vi "myRIO_BRig_Host_formatData_test2.vi"(7 "input_filePath":string, 8 "input_error":errorcluster, 9 "input_data":u16[][](array[numeric]), 10 "input_headers":string[](array[string]), 11 "input_hdl_Workbooks":refnum<k7>) -> (0 "output_error":errorcluster, 3 "output_hdl_Worksbooks":refnum<k7>)   [LabVIEW 2014]
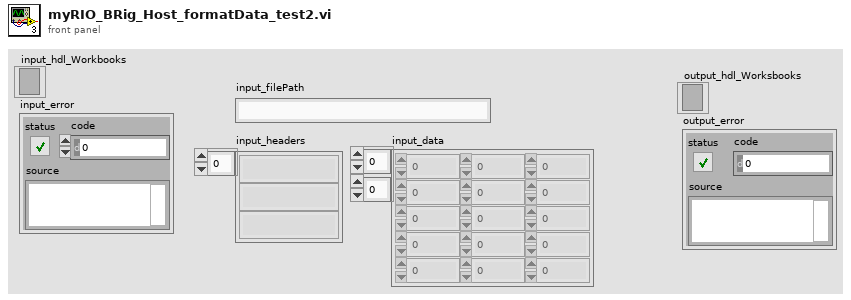
[diagram p1: front panel]
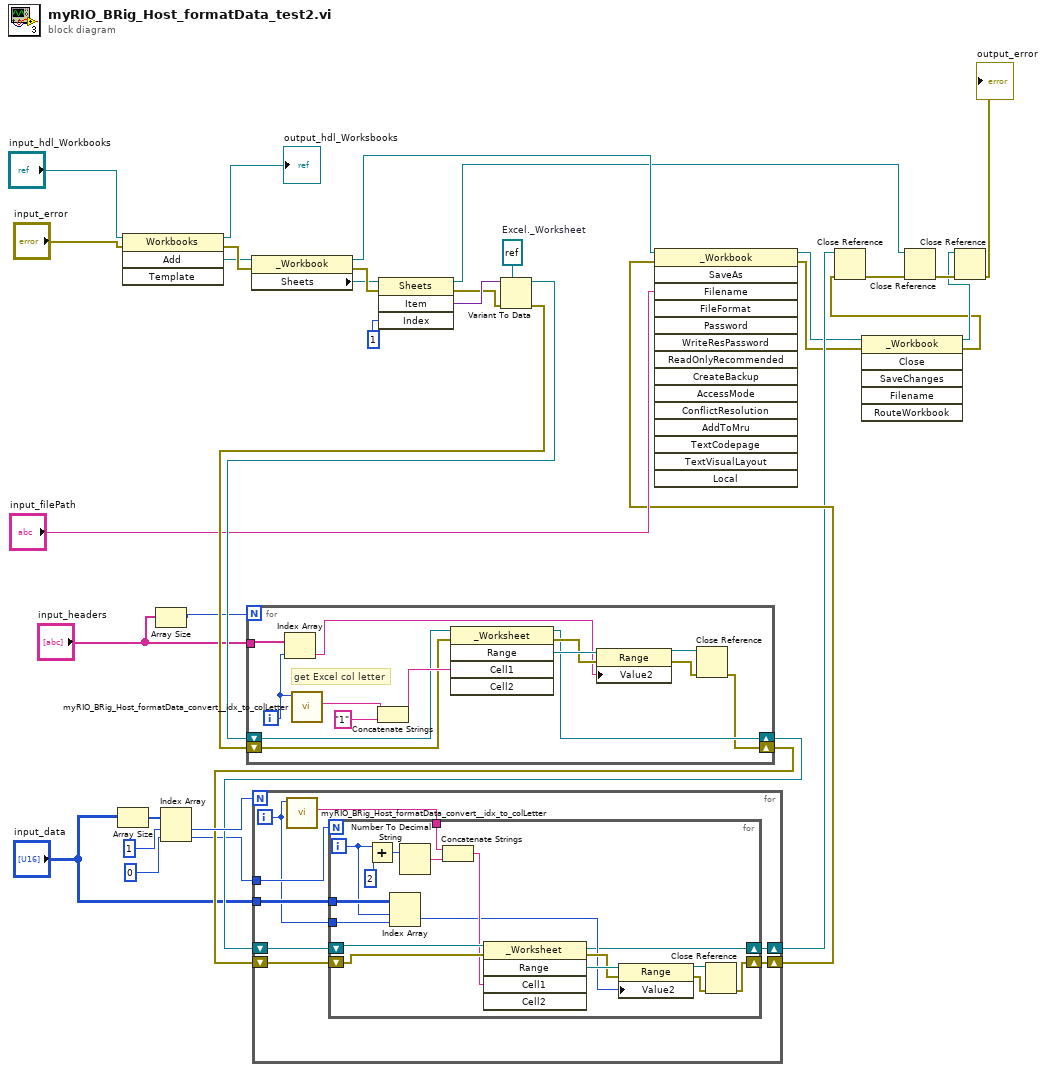
[diagram p0: block diagram]
diagram:
  w30 = refnum<k7> refnum  # Excel._Worksheet
  n1 = Array Size(array="input_data") -> (size(s)=w18:i32[])
  n2 = invoke class="Workbooks" method="Add"(reference="input_hdl_Workbooks", error in="input_error") -> (reference out=→"output_hdl_Worksbooks":refnum<k7>, error out=w34:errorcluster, "Add"=w32:refnum<k7>)  [unwired: 2 in, 1 out]
  n3 = Array Size(array="input_headers") -> (size(s)=w19:i32)
  n4 = Index Array(array=w18, index #1=1 ("index"), index #2=0 ("index")) -> (element #1=w15:i32, element #2=w12:i32)
  n5 = property class="_Workbook"(reference=w32, error in=w34) -> (reference out=w27:refnum<k7>, error out=w35:errorcluster, "Sheets"=w31:refnum<k7>)
  n6 = invoke class="Sheets" method="Item"(reference=w31, error in=w35, "Index"=1) -> (reference out=w26:refnum<k7>, error out=w28:errorcluster, "Item"=w29:variant)  [unwired: 1 in, 1 out]
  n7 = Variant To Data(error in=w28, type=w30, Variant=w29) -> (data=w22:refnum<k7>, error out=w23:errorcluster)
  n8 = for {
    N: w19 -> [_]
    tunnel: "input_headers" -> [w49]
    shift-right: [w39] -> w13
    shift-left: w22 -> [w41]
    shift-right: [w36] -> w14
    shift-left: w23 -> [w40]
    i -> [w48]
    # "get Excel col letter"
    n9 = Index Array(array=w49, index=w48) -> (element=w42:string)
    n10 = call "myRIO_BRig_Host_formatData_convert__idx_to_colLetter.vi"("input_idx"=w48) -> ("output_colLetter"=w46:string)  [unwired: 10 in]
    n11 = Concatenate Strings(w46, "1" ("string")) -> (w45:string)
    n12 = invoke class="_Worksheet" method="Range"(reference=w41, error in=w40, "Cell1"=w45) -> (reference out=w39:refnum<k7>, error out=w43:errorcluster, "Range"=w44:refnum<k7>)  [unwired: 2 in, 2 out]
    n13 = property class="Range"(reference=w44, error in=w43, "Value2"=w42) -> (reference out=w38:refnum<k7>, error out=w37:errorcluster)
    n14 = Close Reference(reference=w38, error in (no error)=w37) -> (error out=w36:errorcluster)
  }
  n15 = for {
    N: w15 -> [_]
    shift-right: [w51] -> w10
    shift-left: w14 -> [w57]
    shift-right: [w50] -> w9
    shift-left: w13 -> [w56]
    tunnel: w12 -> [w55]
    tunnel: "input_data" -> [w53]
    i -> [w52]
    n16 = call "myRIO_BRig_Host_formatData_convert__idx_to_colLetter.vi"("input_idx"=w52) -> ("output_colLetter"=w54:string)  [unwired: 10 in]
    n17 = for {
      N: w55 -> [_]
      shift-right: [w59] -> w51
      shift-left: w57 -> [w66]
      shift-right: [w58] -> w50
      shift-left: w56 -> [w67]
      tunnel: w54 -> [w71]
      tunnel: w53 -> [w70]
      tunnel: w52 -> [w68]
      i -> [w69]
      n18 = Add(x=w69, y=2 ("string")) -> (x+y=w73:i32)
      n19 = Index Array(array=w70, index (row)=w69, index (col)=w68) -> (element=w62:u16)
      n20 = Number To Decimal String(number=w73) -> (decimal integer string=w72:string)  [unwired: 1 in]
      n21 = Concatenate Strings(w71, w72) -> (w65:string)
      n22 = invoke class="_Worksheet" method="Range"(reference=w67, error in=w66, "Cell1"=w65) -> (reference out=w58:refnum<k7>, error out=w63:errorcluster, "Range"=w64:refnum<k7>)  [unwired: 2 in, 2 out]
      n23 = property class="Range"(reference=w64, error in=w63, "Value2"=w62) -> (reference out=w61:refnum<k7>, error out=w60:errorcluster)
      n24 = Close Reference(reference=w61, error in (no error)=w60) -> (error out=w59:errorcluster)
    }
  }
  n25 = invoke class="_Workbook" method="SaveAs"(reference=w27, error in=w10, "Filename"="input_filePath") -> (reference out=w3:refnum<k7>, error out=w4:errorcluster)  [unwired: 12 in, 13 out]
  n26 = invoke class="_Workbook" method="Close"(reference=w3, error in=w4) -> (reference out=w2:refnum<k7>, error out=w1:errorcluster)  [unwired: 4 in, 4 out]
  n27 = Close Reference(reference=w9, error in (no error)=w1) -> (error out=w25:errorcluster)
  n28 = Close Reference(reference=w26, error in (no error)=w25) -> (error out=w24:errorcluster)
  n29 = Close Reference(reference=w2, error in (no error)=w24) -> (error out=→"output_error":errorcluster)
